vi "ADFX_Ensure_Save.vi"(8 "error in (no error)":errorcluster, 11 "Data in":T1) -> (0 "error out":errorcluster, 3 "Data out":T1)   [LabVIEW 2015]
doc: "Checks if control data has been saved, prompts to save or continue."
uses:
  controls/AFXP Data.ctl
  controls/AFCP Setup.ctl
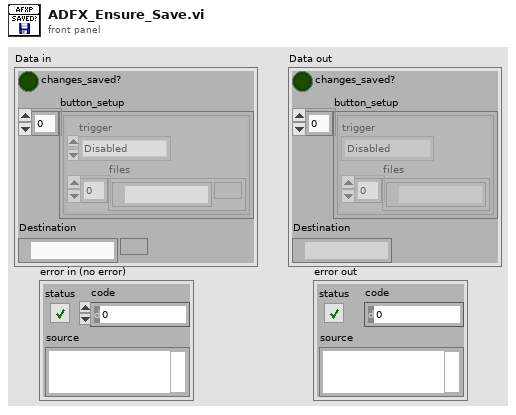
[diagram p1: front panel]
types:
  T1 = typedef "AFXP Data.ctl" = cluster{"changes_saved?":bool, "button_setup":T2[], "Destination":path}
  T2 = typedef "AFCP Setup.ctl" = cluster{"trigger":enum16{"Basic", "Hold-Loop", "Latch-Loop", "Next", "Random", "Disabled"}, "files":path[]}
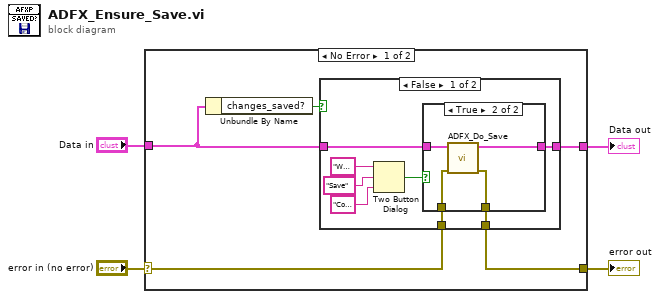
[diagram p0: block diagram]
diagram:
  n1 = case shown="No Error" "error in (no error)" {
    selector: "error in (no error)" -> [w5 w27]
    tunnel: [w9 w26] -> w4
    tunnel: "Data in" -> [w8 w26]
    tunnel: [w7 w27] -> w2
    frame No Error {
      n2 = Unbundle By Name(w8) -> ("changes_saved?"=w6:bool)
      n3 = case shown="False" w6 {
        tunnel: w5 -> [w13 w24]
        tunnel: [w12 w24] -> w7
        tunnel: w8 -> [w11 w25]
        tunnel: [w10 w25] -> w9
        frame False {
          n4 = Two Button Dialog(message="Warning: Project not saved", 1:"Continue without Saving" ("message"), 2:"Save" ("message")) -> (T button?=w16:bool)
          n5 = case shown="True" w16 {
            tunnel: w13 -> [w18 w23]
            tunnel: [w18 w22] -> w12
            tunnel: w11 -> [w19 w21]
            tunnel: [w19 w20] -> w10
            frame False {
            }
            frame True {
              n6 = call "ADFX_Do_Save.vi"("error in (no error)"=w23, "Data in"=w21) -> ("error out"=w22:errorcluster, "Data out"=w20:T1)  [unwired: 8 in]
            }
          }
        }
        frame True {
        }
      }
    }
    frame Error {
    }
  }
  "Data out" <- w4
  "error out" <- w2
